vi "Line 1 to End Switch 1.vi"(6 "Command Info In":T2, 7 "Block Inputs":T1, 8 "Position":T5=enum."Far Right") -> (0 "Command Info Out":T2)   [LabVIEW 2017]
uses:
  Support Code/Starting Position.ctl
  <vilib>/Rock Robotics/WPI/Framework/Command Status Info.ctl
  <vilib>/Rock Robotics/WPI/Framework/Completion Status.ctl
  <vilib>/Rock Robotics/WPI/Framework/Completion Notifier.ctl
  Support Code/Extended Block Inputs.ctl
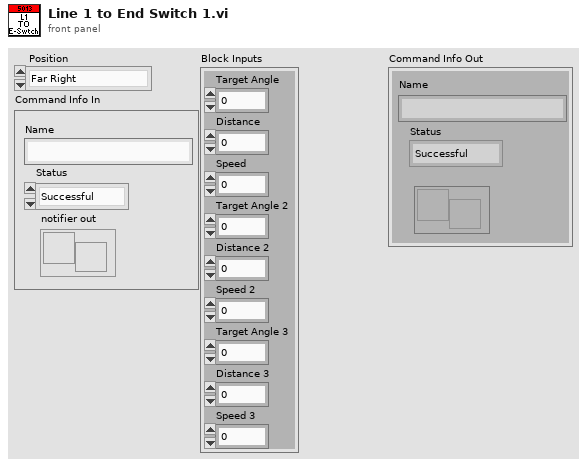
[diagram p1: front panel]
types:
  T1 = typedef "Extended Block Inputs.ctl" = cluster{"Target Angle":dbl, "Distance":dbl, "Speed":dbl, "Target Angle 2":dbl, "Distance 2":dbl, "Speed 2":dbl, "Target Angle 3":dbl, "Distance 3":dbl, "Speed 3":dbl}
  T2 = typedef "Command Status Info.ctl" = cluster{"Name":string, "Status":T3, "notifier out":T4}
  T3 = typedef "Completion Status.ctl" = enum16{"Successful", "Aborted", "Incomplete"}
  T4 = typedef "Completion Notifier.ctl" = refnum<notifier>
  T5 = typedef "Starting Position.ctl" = enum16{"Far Left", "Center", "Far Right"}
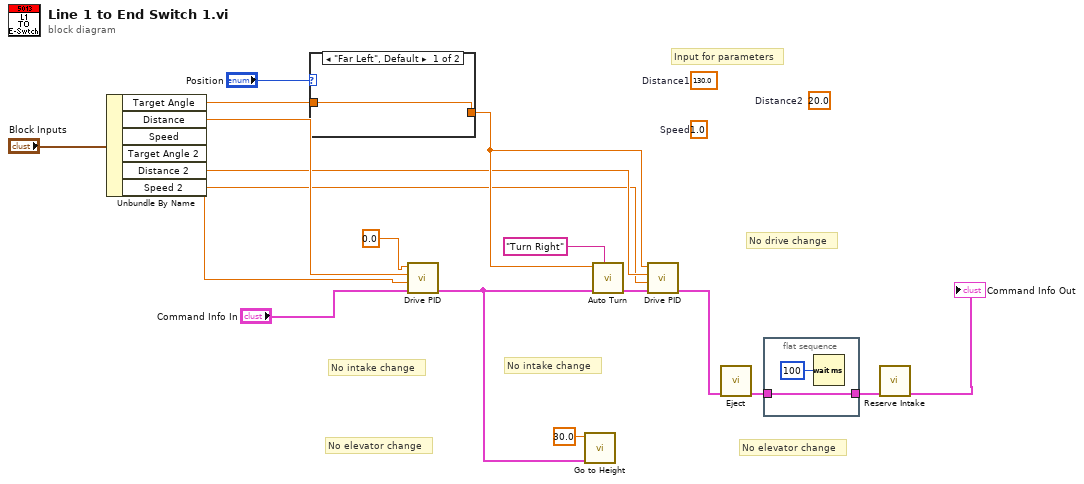
[diagram p0: block diagram]
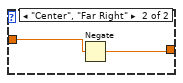
[diagram p2: hidden frame]
diagram:
  (unwired) 20.0  # Distance2
  (unwired) 1.0  # Speed
  (unwired) 130.0  # Distance1
  # "Input for parameters"
  # "No drive change"
  # "No elevator change"
  # "No intake change"
  # "No intake change"
  # "No elevator change"
  n1 = Unbundle By Name("Block Inputs") -> ("Target Angle"=w8:dbl, "Distance"=w5:dbl, "Speed"=w3:dbl, "Distance 2"=w2:dbl, "Speed 2"=w1:dbl)  [unwired: 1 out]
  n2 = case shown="\"Far Left\", Default" "Position" {
    tunnel: [w19 w21] -> w10
    tunnel: w8 -> [w19 w20]
    frame "Far Left", Default {
    }
    frame "Center", "Far Right" {
      n3 = Negate(x=w20) -> (-x=w21:dbl)
    }
  }
  n4 = call "Drive PID.vi"("Command Info In"="Command Info In", "Speed"=w3, "Distance"=w5, "Target Angle"=0.0 ("Distance")) -> ("Command Info Out"=w12:T2)  [unwired: 7 in]
  n5 = call "Go to Height.vi"("Command Info In"=w12, "Target Height (in)"=30.0) -> ()  [unwired: 9 in, 1 out]
  n6 = call "Auto Turn.vi"("Description"="Turn Right", "Command Info In"=w12, "Target Angle"=w10) -> ("Command Info Out"=w13:T2)  [unwired: 8 in]
  n7 = call "Drive PID.vi"("Command Info In"=w13, "Speed"=w1, "Distance"=w2, "Target Angle"=w10) -> ("Command Info Out"=w16:T2)  [unwired: 7 in]
  n8 = call "Eject.vi"("Command Info In"=w16) -> ("Command Info Out"=w17:T2)  [unwired: 10 in]
  n9 = flat-sequence {
    tunnel: w17 -> [w23]
    tunnel: [w23] -> w11
    frame #0 {
      n10 = Wait (ms)(milliseconds to wait=u32 100) -> ()  [unwired: 1 out]
    }
  }
  n11 = call "Reserve Intake.vi"("Command Info"=w11) -> ("Command Info"=→"Command Info Out":T2)  [unwired: 10 in]
